vi "SENS_IF_FILT_SAMP_PER_MODE.vi"(0 "VISA IN":refnum<visa-resource-name>, 1 "Mode":string, 5 "error in":errorcluster, 7 "Channel":i32) -> (14 "VISA Out":refnum<visa-resource-name>, 19 "error out":errorcluster)   [LabVIEW 2018, in "PNA-X.lvlib"]
doc: "SENSe<cnum>:IF:FILTer:SAMPle:PERiod:MODE <char> \n(Read-Write) Sets and returns the IF filter sample period mode to the specified value. Critical Note: \nParameters \n<cnum> Existing channel number to manipulate. If unspecified, <cnum> is set to 1. \n<char> Sample period mode. Choose from AUTO or MANUAL. \nExamples SENS:IF:FILT:SAMP:PER:MODE MANUAL \nsense2:if:filter:sample:period:mode AUTO \nQuery Syntax SENS:IF:FILTer:SAMPle:PERiod:MODE? \nReturn Type Character \nDefault AUTO"
uses:
  PNA-X.lvlib
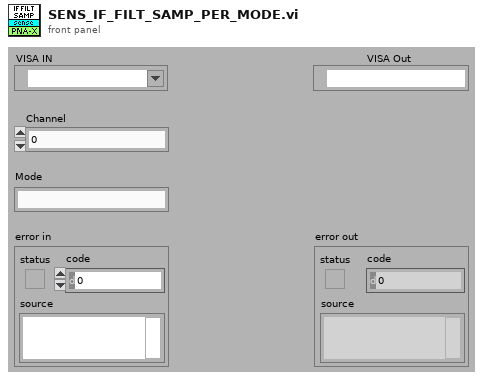
[diagram p1: front panel]
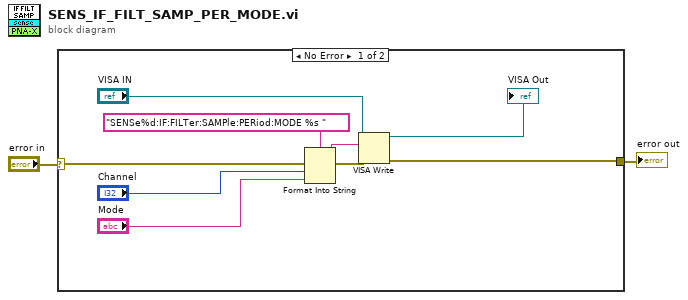
[diagram p0: block diagram]
diagram:
  n1 = case shown="No Error" "error in" {
    selector: "error in" -> [w11 w12]
    tunnel: [w4 w12] -> w1
    frame No Error {
      n2 = Format Into String(format string="SENSe%d:IF:FILTer:SAMPle:PERiod:MODE %s " ("Cmdline"), error in=w11, "Channel", "Mode") -> (resulting string=w9:string, error out=w10:errorcluster)  [unwired: 1 in]
      n3 = VISA Write(VISA resource name="VISA IN", write buffer=w9, error in (no error)=w10) -> (VISA resource name out=→"VISA Out":refnum<visa-resource-name>, error out=w4:errorcluster)  [unwired: 1 out]
    }
    frame Error {
    }
  }
  "error out" <- w1
